vi "Build Shared Library Search Path.vi"(8 "Error In":errorcluster, 11 "labssh2 Shared Library":path=path "") -> (0 "Error Out":errorcluster, 3 "Search Path":path[](array[path]))   [LabVIEW 2017, in "LabSSH2.lvlib"]
uses:
  LabSSH2.lvlib
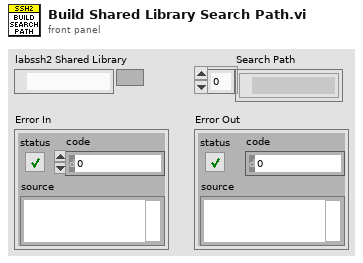
[diagram p1: front panel]
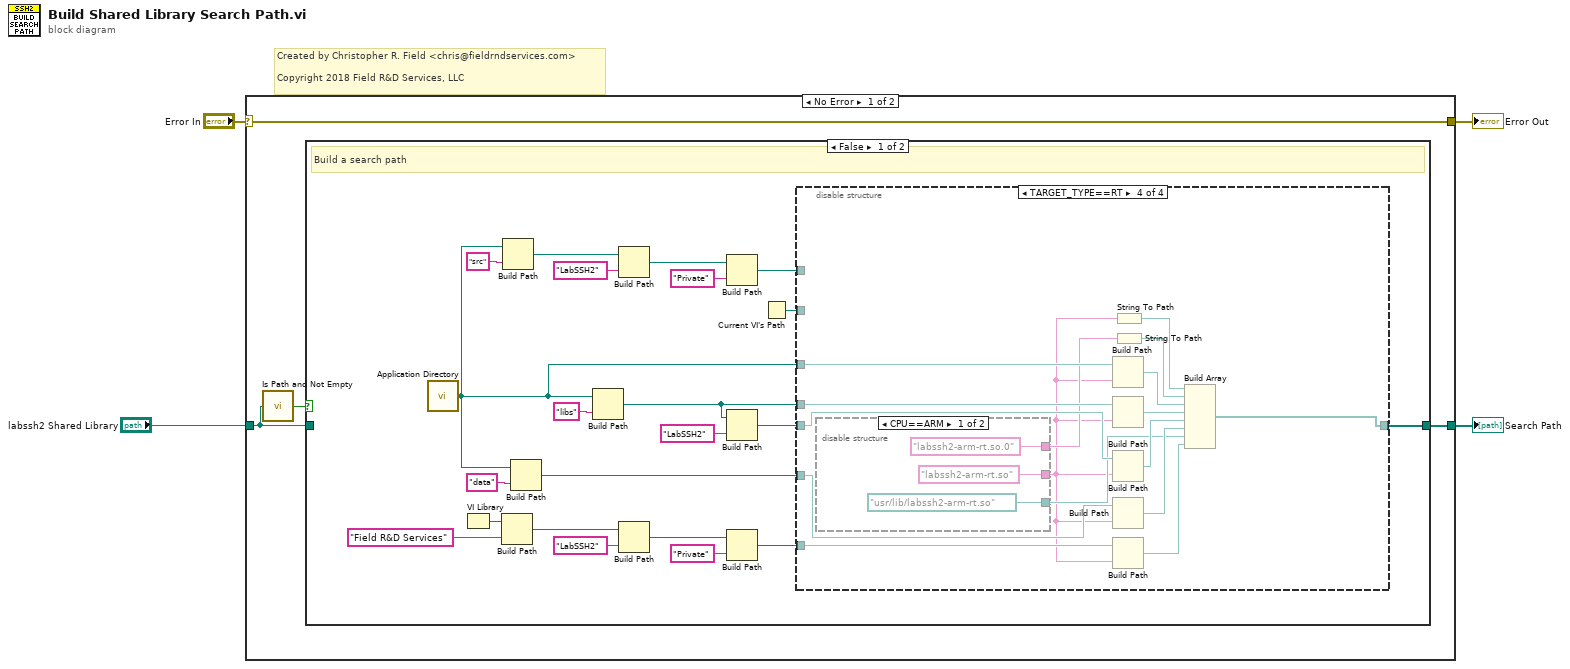
[diagram p0: block diagram]
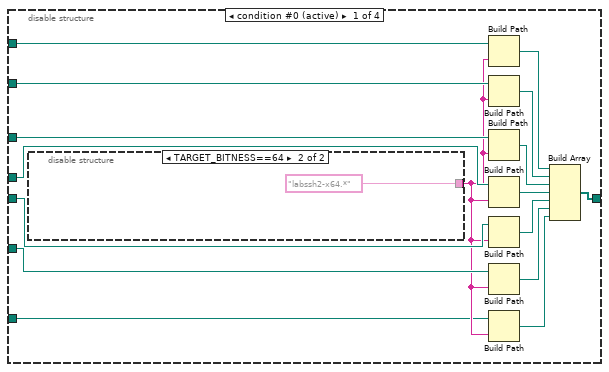
[diagram p2: hidden frame]
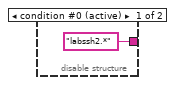
[diagram p3: hidden frame]
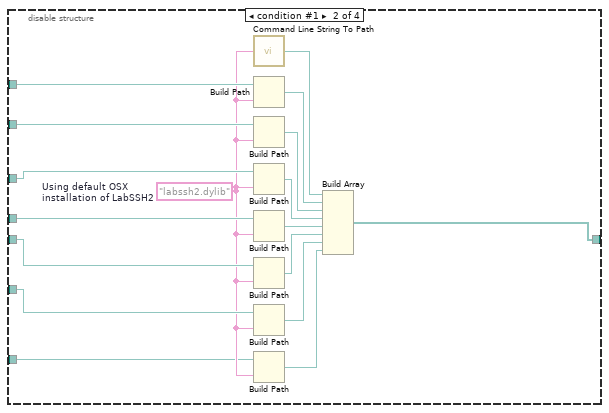
[diagram p4: hidden frame]
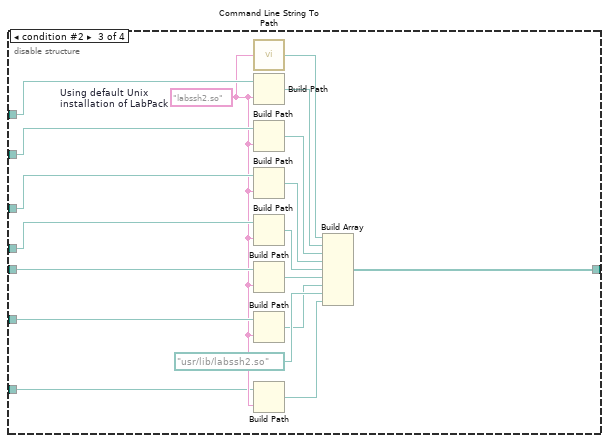
[diagram p5: hidden frame]
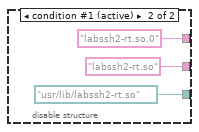
[diagram p6: hidden frame]
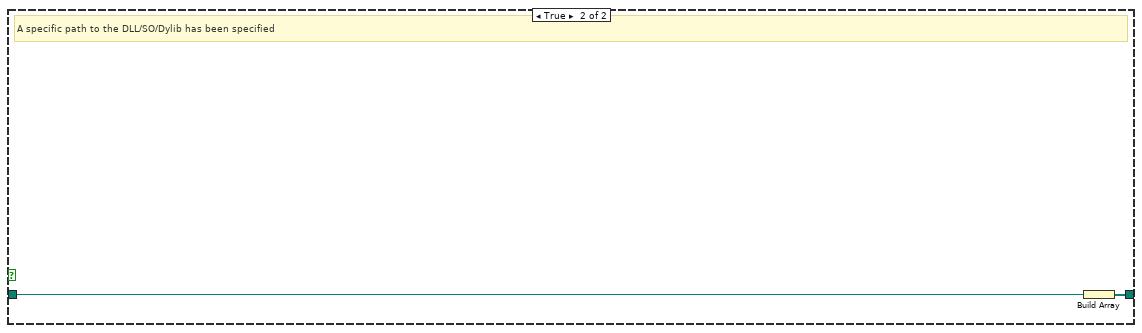
[diagram p7: hidden frame]
diagram:
  # "Created by Christopher R. Field <chris@fieldrndservices.com>\n\nCopyright 2018 Field R&D Services, LLC"
  n1 = case shown="No Error" "Error In" {
    selector: "Error In" -> [w5 w108]
    tunnel: [w8 _] -> w4
    tunnel: "labssh2 Shared Library" -> [w7 _]
    tunnel: [w5 w108] -> w1
    frame No Error {
      n2 = call <vilib>:"Is Path and Not Empty.vi"("path"=w7) -> ("Is Path and Not Empty?"=w6:bool)  [unwired: 4 in]
      n3 = case shown="False" w6 {
        tunnel: w7 -> [_ w107]
        tunnel: [w23 w106] -> w8
        frame False {
          # "Build a search path"
          n4 = call <vilib>:"Application Directory.vi"() -> ("Application Directory"=w21:path)
          n5 = VI Library() -> (path=w15:path)
          n6 = Build Path(base path=w15, name or relative path="Field R&D Services") -> (appended path=w13:path)
          n7 = Build Path ("EXE include\nlocation")(base path=w21, name or relative path="src") -> (appended path=w27:path)
          n8 = Build Path ("EXE include\nlocation")(base path=w21, name or relative path="data") -> (appended path=w19:path)
          n9 = Build Path ("EXE include\nlocation")(base path=w21, name or relative path="libs") -> (appended path=w18:path)
          n10 = Build Path ("EXE include\nlocation")(base path=w27, name or relative path="LabSSH2") -> (appended path=w29:path)
          n11 = Build Path(base path=w13, name or relative path="LabSSH2") -> (appended path=w11:path)
          n12 = Build Path ("EXE include\nlocation")(base path=w29, name or relative path="Private") -> (appended path=w25:path)
          n13 = Build Path ("EXE include\nlocation")(base path=w18, name or relative path="LabSSH2") -> (appended path=w16:path)
          n14 = Build Path(base path=w11, name or relative path="Private") -> (appended path=w9:path)
          n15 = Current VI's Path() -> (path=w24:path)
          n16 = disable-structure shown="TARGET_TYPE==RT" {
            disable-tunnel: [w43 w64 w82 w99] -> w23
            disable-tunnel: w25 -> [w46 w63 w81 _]
            disable-tunnel: w24 -> [w45 w61 w79 _]
            disable-tunnel: w21 -> [w41 w59 w72 w92]
            disable-tunnel: w18 -> [w39 w58 w71 w91]
            disable-tunnel: w19 -> [w38 w56 w69 w89]
            disable-tunnel: w16 -> [w35 w57 w70 w90]
            disable-tunnel: w9 -> [w32 w50 w67 w86]
            frame condition #0 (active) {
              n17 = disable-structure shown="TARGET_BITNESS==64" {
                disable-tunnel: ["labssh2.*" ("name or relative path") "labssh2-x64.*" ("name or relative path")] -> w33
                frame condition #0 (active) {
                }
                frame condition #1 {
                }
              }
              n18 = Build Path ("EXE include\nlocation")(base path=w46, name or relative path=w33) -> (appended path=w44:path)
              n19 = Build Path ("EXE include\nlocation")(base path=w45, name or relative path=w33) -> (appended path=w42:path)
              n20 = Build Path ("EXE include\nlocation")(base path=w41, name or relative path=w33) -> (appended path=w40:path)
              n21 = Build Path ("EXE include\nlocation")(base path=w39, name or relative path=w33) -> (appended path=w37:path)
              n22 = Build Path ("EXE include\nlocation")(base path=w35, name or relative path=w33) -> (appended path=w34:path)
              n23 = Build Path ("EXE include\nlocation")(base path=w38, name or relative path=w33) -> (appended path=w36:path)
              n24 = Build Path ("EXE include\nlocation")(base path=w32, name or relative path=w33) -> (appended path=w31:path)
              n25 = Build Array(w44, w42, w40, w37, w34, w36, w31) -> (w43:path[])
            }
            frame condition #1 {
              w51 = "labssh2.dylib"  # Using default OSX installation of LabSSH2
              n26 = call <vilib>:"Command Line String To Path.vi"("string"=w51) -> ("path"=w65:path)
              n27 = Build Path ("EXE include\nlocation")(base path=w63, name or relative path=w51) -> (appended path=w62:path)
              n28 = Build Path ("EXE include\nlocation")(base path=w61, name or relative path=w51) -> (appended path=w60:path)
              n29 = Build Path ("EXE include\nlocation")(base path=w59, name or relative path=w51) -> (appended path=w55:path)
              n30 = Build Path ("EXE include\nlocation")(base path=w58, name or relative path=w51) -> (appended path=w54:path)
              n31 = Build Path ("EXE include\nlocation")(base path=w57, name or relative path=w51) -> (appended path=w53:path)
              n32 = Build Path ("EXE include\nlocation")(base path=w56, name or relative path=w51) -> (appended path=w52:path)
              n33 = Build Path ("EXE include\nlocation")(base path=w50, name or relative path=w51) -> (appended path=w49:path)
              n34 = Build Array(w65, w62, w60, w55, w54, w53, w52, w49) -> (w64:path[])
            }
            frame condition #2 {
              w68 = "labssh2.so"  # Using default Unix installation of LabPack
              n35 = call <vilib>:"Command Line String To Path.vi"("string"=w68) -> ("path"=w83:path)
              n36 = Build Path ("EXE include\nlocation")(base path=w81, name or relative path=w68) -> (appended path=w80:path)
              n37 = Build Path ("EXE include\nlocation")(base path=w79, name or relative path=w68) -> (appended path=w78:path)
              n38 = Build Path ("EXE include\nlocation")(base path=w72, name or relative path=w68) -> (appended path=w76:path)
              n39 = Build Path ("EXE include\nlocation")(base path=w71, name or relative path=w68) -> (appended path=w75:path)
              n40 = Build Path ("EXE include\nlocation")(base path=w70, name or relative path=w68) -> (appended path=w74:path)
              n41 = Build Path ("EXE include\nlocation")(base path=w69, name or relative path=w68) -> (appended path=w73:path)
              n42 = Build Path ("EXE include\nlocation")(base path=w67, name or relative path=w68) -> (appended path=w66:path)
              n43 = Build Array(w83, w80, w78, w76, w75, w74, w73, path "/usr/lib/labssh2.so" ("path"), w66) -> (w82:path[])
            }
            frame condition #3 {
              n44 = disable-structure shown="CPU==ARM" {
                disable-tunnel: ["labssh2-arm-rt.so.0" "labssh2-rt.so.0"] -> w88
                disable-tunnel: ["labssh2-arm-rt.so" "labssh2-rt.so"] -> w85
                disable-tunnel: [path "/usr/lib/labssh2-arm-rt.so" ("path") path "/usr/lib/labssh2-rt.so" ("path")] -> w87
                frame condition #0 {
                }
                frame condition #1 (active) {
                }
              }
              n45 = Build Path ("EXE include\nlocation")(base path=w92, name or relative path=w85) -> (appended path=w93:path)
              n46 = Build Path ("EXE include\nlocation")(base path=w91, name or relative path=w85) -> (appended path=w96:path)
              n47 = Build Path ("EXE include\nlocation")(base path=w90, name or relative path=w85) -> (appended path=w95:path)
              n48 = Build Path ("EXE include\nlocation")(base path=w89, name or relative path=w85) -> (appended path=w94:path)
              n49 = Build Path ("EXE include\nlocation")(base path=w86, name or relative path=w85) -> (appended path=w84:path)
              n50 = String To Path(string=w85) -> (path=w98:path)
              n51 = String To Path(string=w88) -> (path=w97:path)
              n52 = Build Array(w98, w97, w93, w96, w95, w94, w87, w84) -> (w99:path[])
            }
          }
        }
        frame True {
          # "A specific path to the DLL/SO/Dylib has been specified"
          n53 = Build Array(w107) -> (w106:path[])
        }
      }
    }
    frame Error {
    }
  }
  "Search Path" <- w4
  "Error Out" <- w1
